vi "nextSiblingNode.vi"(8 "error in (no error)":errorcluster caption="errorIn", 11 "siblingNode":refnum<k20>) -> (0 "error out":errorcluster caption="errorOut", 2 "found?":bool caption="found？", 3 "siblingNode":refnum<k20>)   [LabVIEW 2017]
uses:
  <vilib>/xml/Close Reference(Node).vi
  <vilib>/xml/NI_XML.lvlib
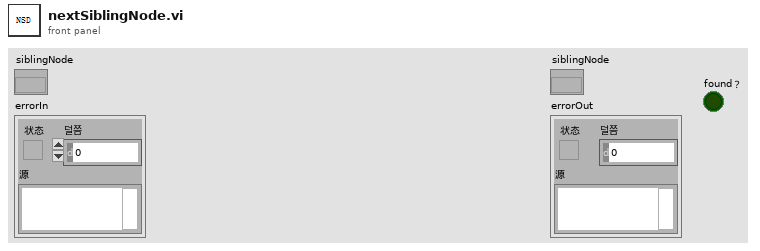
[diagram p1: front panel]
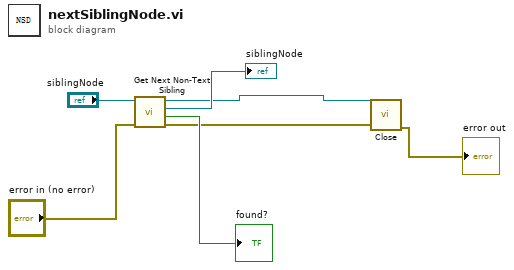
[diagram p0: block diagram]
diagram:
  n1 = call <vilib>:"Get Next Non-Text Sibling.vi"("error in (no error)"="error in (no error)", "node in"="siblingNode") -> ("error out"=w2:errorcluster, "found sibling node?"=→"found?":bool, "sibling node"=→"siblingNode":refnum<k20>, "node out"=w3:refnum<k20>)  [unwired: 6 in]
  n2 = call-poly <vilib>:"Close.vi"("error in (no error)"=w2, "node"=w3) -> ("error out"=→"error out":errorcluster)  [unwired: 7 in]
